vi "RequestsJasonToArray.vi"(8 "error in (no error)":errorcluster, 11 "Data Out":string) -> (0 "error out":errorcluster, 3 "REQs":string[](array[string]))   [LabVIEW 2015]
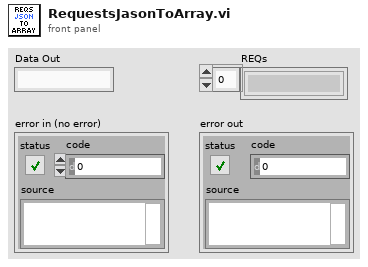
[diagram p1: front panel]
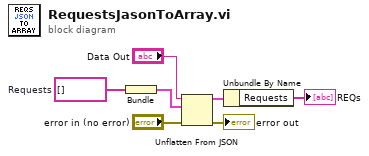
[diagram p0: block diagram]
diagram:
  w3 = string[] []  # Requests
  n1 = Bundle("Requests"=w3) -> (w2:cluster{"Requests":string[]})  [unwired: 1 in]
  n2 = Unflatten From JSON(JSON string="Data Out", type and defaults=w2, error in (no error)="error in (no error)") -> (value=w1:cluster{"Requests":string[]}, error out=→"error out":errorcluster)  [unwired: 4 in]
  n3 = Unbundle By Name(w1) -> ("Requests"=→"REQs":string[])
